vi "Normalise Inlet Temps array.vi"(1 "Temps plus setpoints":dbl[](array[numeric]) format="%.2f") -> (0 "Normalised Temps":dbl[](array[numeric]))   [LabVIEW 2013]
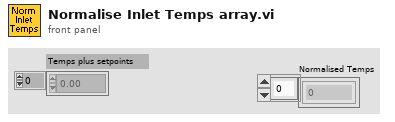
[diagram p1: front panel]
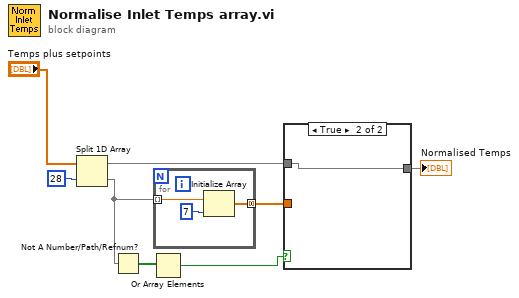
[diagram p0: block diagram]
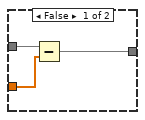
[diagram p2: hidden frame]
diagram:
  n1 = Split 1D Array(array="Temps plus setpoints", index=28) -> (first subarray=w5:dbl[], second subarray=w4:dbl[])
  n2 = Not A Number/Path/Refnum?(number/path/refnum=w4) -> (NaN/Path/Refnum?=w3:bool[])
  n3 = Or Array Elements(Boolean array=w3) -> (logical OR=w2:bool)
  n4 = for {
    tunnel: w4 -> [w10] mode=indexing
    tunnel: [w9] -> w6 mode=concatenating
    n5 = Initialize Array(w10, 7 ("dimension size")) -> (w9:dbl[])
  }
  n6 = case shown="True" w2 {
    tunnel: w6 -> [w14 _]
    tunnel: w5 -> [w13 w15]
    tunnel: [w12 w15] -> w1
    frame False {
      n7 = Subtract(x=w13, y=w14) -> (x-y=w12:dbl[])
    }
    frame True {
    }
  }
  "Normalised Temps" <- w1
